vi "Count Calls.vi"(6 "Comparator in":refnum<class "Comparator.lvclass">, 8 "error in (no error)":errorcluster, 11 "Calls in":refnum<class "VI Server VI Call.lvclass">[](array[class])) -> (0 "error out":errorcluster, 2 "Call Count":i32[](array[numeric]), 3 "Unique Calls":refnum<class "VI Server VI Call.lvclass">[](array[class]))   [LabVIEW 2020, in "One or More.lvclass"]
uses:
  One or More.lvclass
  Framework/VI Server VI Call/VI Server VI Call.lvclass
  Framework/Comparator/Comparator.lvclass
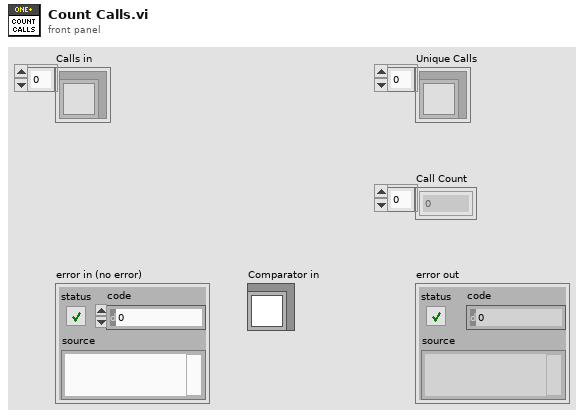
[diagram p1: front panel]
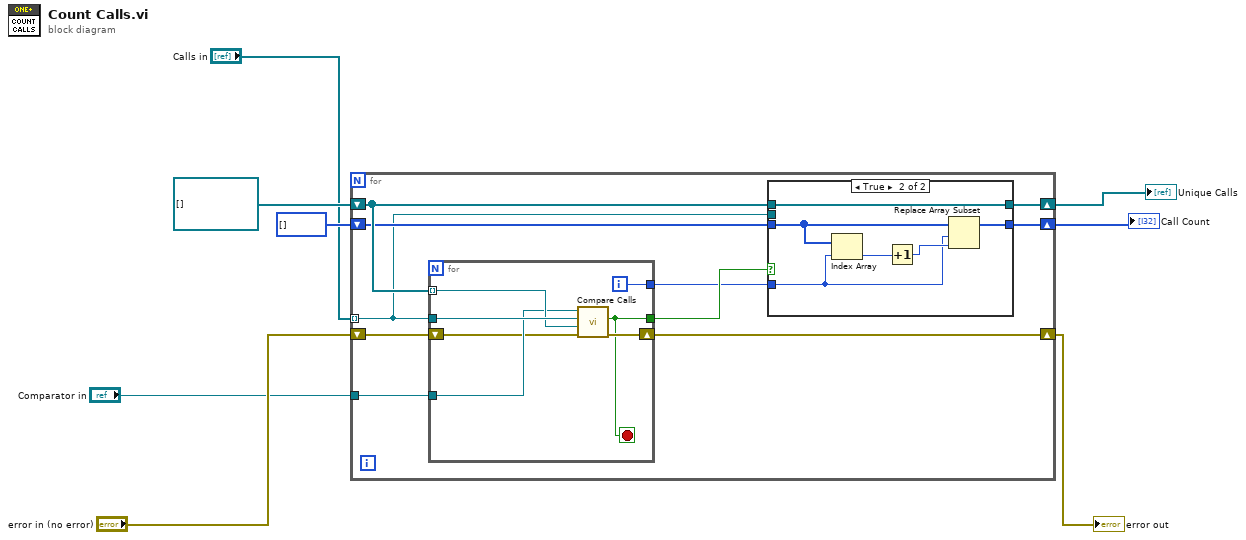
[diagram p0: block diagram]
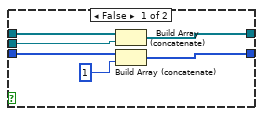
[diagram p2: hidden frame]
diagram:
  n1 = for {
    tunnel: "Calls in" -> [w9] mode=indexing
    shift-right: [w14] -> w7
    shift-left: refnum<class "VI Server VI Call.lvclass">[] [] -> [w15]
    tunnel: "Comparator in" -> [w18]
    shift-right: [w16] -> w4
    shift-left: "error in (no error)" -> [w17]
    shift-right: [w11] -> w8
    shift-left: i32[] [] -> [w12]
    n2 = for {
      tunnel: w9 -> [w37]
      tunnel: w15 -> [w36] mode=indexing
      tunnel: w18 -> [w35]
      shift-right: [w33] -> w16
      shift-left: w17 -> [w34]
      tunnel: [w32] -> w13
      tunnel: [w31] -> w10
      i -> [w31]
      stop <- w32 stop-if-true
      n3 = call-dynamic "Compare Calls.vi"("error in (no error)"=w34, "VI Call 2"=w36, "VI Call 1"=w37, "Comparator in"=w35) -> ("error out"=w33:errorcluster, "Equal?"=w32:bool)  [unwired: 5 in, 1 out]
    }
    n4 = case shown="True" w13 {
      tunnel: w15 -> [w24 w30]
      tunnel: [w22 w30] -> w14
      tunnel: w12 -> [w23 w29]
      tunnel: [w20 w28] -> w11
      tunnel: w10 -> [_ w25]
      tunnel: w9 -> [w21 _]
      frame False {
        n5 = Build Array (concatenate)(w24, w21) -> (w22:refnum<class "VI Server VI Call.lvclass">[])
        n6 = Build Array (concatenate)(w23, 1) -> (w20:i32[])
      }
      frame True {
        n7 = Index Array(array=w29, index=w25) -> (element=w27:i32)
        n8 = Increment(x=w27) -> (x+1=w26:i32)
        n9 = Replace Array Subset(array=w29, new element=w26, index=w25) -> (w28:i32[])
      }
    }
  }
  "Call Count" <- w8
  "Unique Calls" <- w7
  "error out" <- w4
